vi "Dashboard Main.vi"() -> ()   [LabVIEW 2015]
uses:
  <vilib>/Utility/miscctls.llb/LVRowAndColumnTypeDef.ctl
  <vilib>/event_ctls.llb/eventvkey.ctl
  <vilib>/Rock Robotics/WPI/Dashboard/WPI_DashboardLogging Global.vi
  <vilib>/Rock Robotics/Network Tables/NT Read Numeric Array.vi
  <vilib>/Utility/config.llb/Write Key (String).vi
  <vilib>/Utility/config.llb/Write Key (I32).vi
  <vilib>/Utility/config.llb/NI_LVConfig.lvlib
panel:
  in  "TCP":refnum<k5>
  in  "Rec Mode":enum32{"Stop", "Record", "Playback"}(radio)
  in  "Vision":u16(ring) items=["Camera Off", "USB Camera SW", "USB Camera HW", "IP Camera"]
  out "Camera IP":string
  out "Image Message":string="Timeout in Camera Communications"
  in  "Dashboard Tab":T1(tab)
  out "Speed Control":dbl(slide) scale=0.0..1.0
  out "Right Encoder":dbl format="%#_3g"
  out "Left Encoder":dbl format="%#_3g"
  in  "Autonomous Selection":string(combo)
  out "NT Connection":bool
  in  "Camera Settings":T2={"Frame Rate"=30, "Compression"=30, "Size"=1} {"Frame Rate" scale=1.0..30.0; "Size" items=["640x480", "320x240", "160x120"]}
  out "MotorChart R":cluster{"Numeric":dbl, "Numeric":dbl}(graph)
  out "MotorChart L":T3(graph)
  out "MotorSliders R":cluster{"MotorSlide1":dbl, "MotorSlide2":dbl} {"MotorSlide2" scale=-1.0..1.0 scale format="%#_2e"; "MotorSlide1" scale=-1.0..1.0 scale format="%#_2e"}
  out "MotorSliders L":T4 {"MotorSlide4 2" scale=0.0..14.0 scale format="%#_2e"; "MotorSlide2" scale=-1.0..1.0 scale format="%#_2e"; "MotorSlide1" scale=-1.0..1.0 scale format="%#_2e"}
  out "Gyro":dbl(knob) scale=0.0..360.0
  out "JS1 Z":dbl(slide) scale=-1.0..1.0 scale format="%#_2e"
  out "JS1 Graph":cluster{"X":dbl, "Y":dbl}[](graph)
  out "JS1 Buttons":T5
  out "JS2 Z":dbl(slide) scale=-1.0..1.0 scale format="%#_2e"
  out "JS2 Graph":cluster{"X":dbl, "Y":dbl}[](graph)
  out "JS2 Buttons":T5
  out "Mode":T6(ring)=enum."Auto Disabled"
  in  "DB Camera Config":bool
  out "fps":dbl format="%#.1g"
  out "Mbps":dbl format="%#.1g"
  out "Mbps LED":bool
  out "POV Position":dbl format="%#_3g"
  in  "DB/String 9":string
  in  "DB/String 8":string
  in  "DB/String 7":string
  in  "DB/String 6":string
  in  "DB/String 5":string
  in  "DB/String 4":string
  in  "DB/String 3":string
  in  "DB/String 2":string
  in  "DB/String 1":string
  in  "DB/String 0":string
  in  "DB/Slider 0":dbl(slide) scale=0.0..5.0
  in  "DB/Slider 1":dbl(slide) scale=0.0..5.0
  in  "DB/Slider 2":dbl(slide) scale=0.0..5.0
  in  "DB/Slider 3":dbl(slide) scale=0.0..5.0
  out "DB/LED 3":bool
  out "DB/LED 2":bool
  out "DB/LED 1":bool
  out "DB/LED 0":bool
  in  "DB/Button 3":bool
  in  "DB/Button 2":bool
  in  "DB/Button 1":bool
  in  "DB/Button 0":bool caption="New Name"
  in  "Test Slider":dbl(slide) scale=0.0..100.0 scale format="%#_3g"
  in  "On/Off":bool caption="Solenoid"
  in  "Test Name":u16(ring) items=["Select the test to run..."]
  in  "Test Tree":string(tree)
  in  "Motor":cluster{"Value":dbl, "Enable":bool} {"Value" scale=-1.0..1.0 scale format="%#_3g"}
  out "Progress":T7 {"Test Progress" scale=0.0..100.0}
  in  "Rev/Fwd":cluster{"Forward":bool, "Reverse":bool}
  in  "Test Ring":u16(ring) items=["Monochrome", "Color"]
  out "Cmd Status":string
  in  "Execute Command":bool
  in  "Command Params":string[][](table)
  in  "Command Selection":i32(listbox)
  in  "CheckList":i32(listbox)
  out "Tree":string(tree)
  out "Camera Image":T8(plugin-control)
  out "Background":bool
  # "Left"
  # "Front"
  # "Right"
  # "Battery"
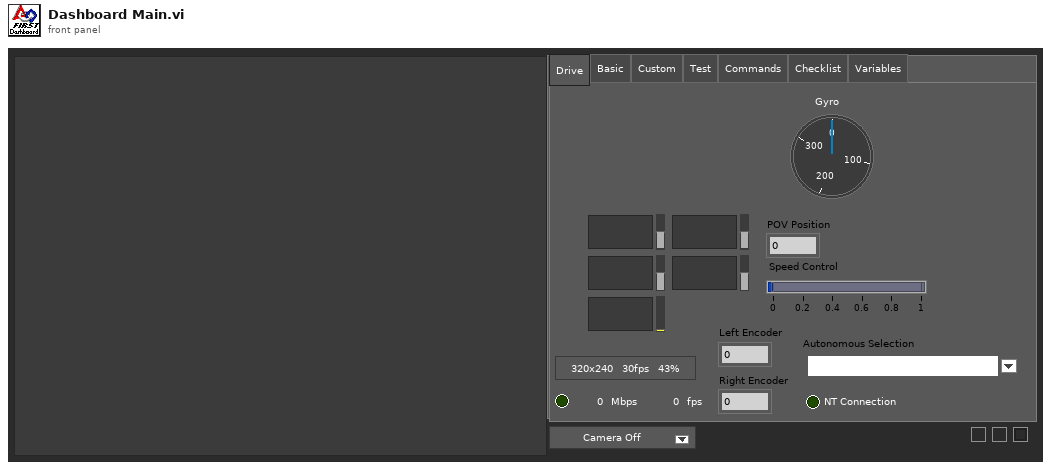
[diagram p1: front panel]
types:
  T1 = enum32{"Drive", "Basic", "Custom", "Test", "Commands", "Checklist", "Variables"}
  T2 = cluster{"Frame Rate":i32, "Compression":i32, "Size":u16}
  T3 = cluster{"Numeric":dbl, "Numeric":dbl, "Battery V":dbl}
  T4 = cluster{"MotorSlide1":dbl, "MotorSlide2":dbl, "MotorSlide4 2":dbl}
  T5 = cluster{bool, bool, bool, bool, bool, bool, bool, bool, bool, bool, bool, bool}
  T6 = enum8{"Tele-Op Disabled", "Tele-Op Enabled", "Auto Disabled", "Auto Enabled", "Test Disabled", "Test Enabled", "Disconnected", "No Code", "E-Stop"}
  T7 = cluster{"Test Progress":u8, "Test Progress Text":string}
  T8 = typedef "IMAQ Image.ctl" = refnum<image>
  T9 = cluster{"IDs":cluster{"RPC field ID":u16, "Unique ID":u16}, "String":string}
  T10 = enum32{"Drive", "Basic", "Custom", "Test", "Checklist", "Variables"}
  T11 = typedef "Image Type" = u32
  T12 = cluster{"Camera Image":refnum<vi>, "Dashboard Tab":refnum<vi>, "Background":refnum<vi>, "Vision":refnum<vi>, "Rec Mode":refnum<vi>, "Test Slider":refnum<vi>, "On/Off ":refnum<vi>, "Test Ring":refnum<vi>, "Rev/Fwd":refnum<vi>, "Test Name":refnum<vi>, "Motor":refnum<vi>, "Progress":refnum<vi>, "CheckList":refnum<vi>, "Tree":refnum<vi>, "Test Tree":refnum<vi>, "Command Params":refnum<vi>, "Command Selection":refnum<vi>, "Execute Command":refnum<vi>, "Cmd Status":refnum<vi>}
  T13 = cluster{"Error Strings":string, "Disable Counts":cluster{u16, u16}, "Rail Faults":cluster{u16, u16, u16}, "Robot IP":string, "DB Mode":u8, "Event Info":cluster{"Name":string, "Type":u8, "Number":u16, "Replay":u8}, "Camera Addr":string}
  T14 = cluster{"Storage":cluster{"Disk Free":u64, "RAM Block":u32, "RAM free":u32}, "CPU Utilization":cluster{"CPU % ISR":sgl, "CPU % Time Crit":sgl, "CPU % Timed Str":sgl, "CPU % High":sgl, "CPU % Above":sgl, "CPU % Normal":sgl, "CPU % Low":sgl}, "CAN":cluster{"% Bus Utilization":sgl, "Bus Off Cnt":u32, "TX_FIFO Full Cnt":u32, "Receive Error Cnt":u8, "Transmit Error Cnt":u8}, "HID":cluster{"HID Outputs":u32, "Rumble Low":u16, "Rumble High":u16}[]}
  T15 = cluster{"Status bits":cluster{"Test Mode":bool, "Autonomous":bool, "Enabled":bool, "Code Start":bool, "Brownout":bool, "Reserved 2":bool, "Reserved 3":bool, "E-Stop":bool}, "Code Trace":cluster{"Disabled":bool, "TeleOp":bool, "Auto":bool, "Test":bool}, "Controller Type":enum16{"unknown", "cRIO", "roboRio"}, "Code?":enum16{"unknown", "noCode", "code"}, "Battery V":dbl}
  T16 = cluster{"Control Bits":cluster{"TestMode":bool, "Autonomous":bool, "Enabled":bool, "FMS Present":bool, bool, bool, bool, "E-Stop":bool}, "Team Station ":u8, "Countdown":sgl, "Joystick Values":cluster{"Axes":dbl[], "Buttons":bool[], "POVs":i16[]}[]}
  T17 = cluster{"Axes":dbl[], "Buttons":bool[], "POVs":i16[]}[]
  T18 = cluster{"Axes":dbl[], "Buttons":bool[], "POVs":i16[]}
  T19 = cluster{"Buttons[0]":bool, "Buttons[1]":bool, "Buttons[2]":bool, "Buttons[3]":bool, "Buttons[4]":bool, "Buttons[5]":bool, "Buttons[6]":bool, "Buttons[7]":bool, "Buttons[8]":bool, "Buttons[9]":bool, "Buttons[10]":bool, "Buttons[11]":bool}
  T20 = typedef "NI_LVConfig.lvlib/Config Data RefNum.ctl" = refnum<k1>
  T21 = cluster{"Operation":enum16{"Update", "Clear"}, "Color Box":u32}[]
  T22 = typedef "eventvkey.ctl" = enum16{"ASCII", "Enter", "Return", "Shift", "Ctrl", "Alt", "Cmd", "Opt", "Caps", "NumLock", "Clear", "Break", "Up", "Down", "Left", "Right", "Insert", "Delete", "Home", "End", "PageUp", "PageDown", "Escape", "Help", "Pause", "ScrollLock", "F1", "F2", "F3", "F4", "F5", "F6", "F7", "F8", "F9", "F10", "F11", "F12", "F13", "F14", "F15", "F16", "F17", "F18", "F19", "F20", "F21", "F22", "F23", "F24", "Play", "VolumeUp", "VolumeDown", "Mute", "Two Byte Char"}
  T23 = cluster{"Image Size":bool, "Image Type":bool, "Pixel Value":bool, "ROI Information":bool, "Zoom Factor":bool}
  T24 = enum8{"Enabled", "Disabled", "Disabled and Grayed Out"}
  T25 = cluster{"Operation":enum16{"Update", "Clear"}, "Color Box":u32}
  T26 = typedef "LVRowAndColumnTypeDef.ctl" = cluster{"Row":i32, "Column":i32}
  T27 = cluster{"Shift":bool, "Ctrl":bool, "Alt":bool, "Cmd":bool, "Opt":bool}
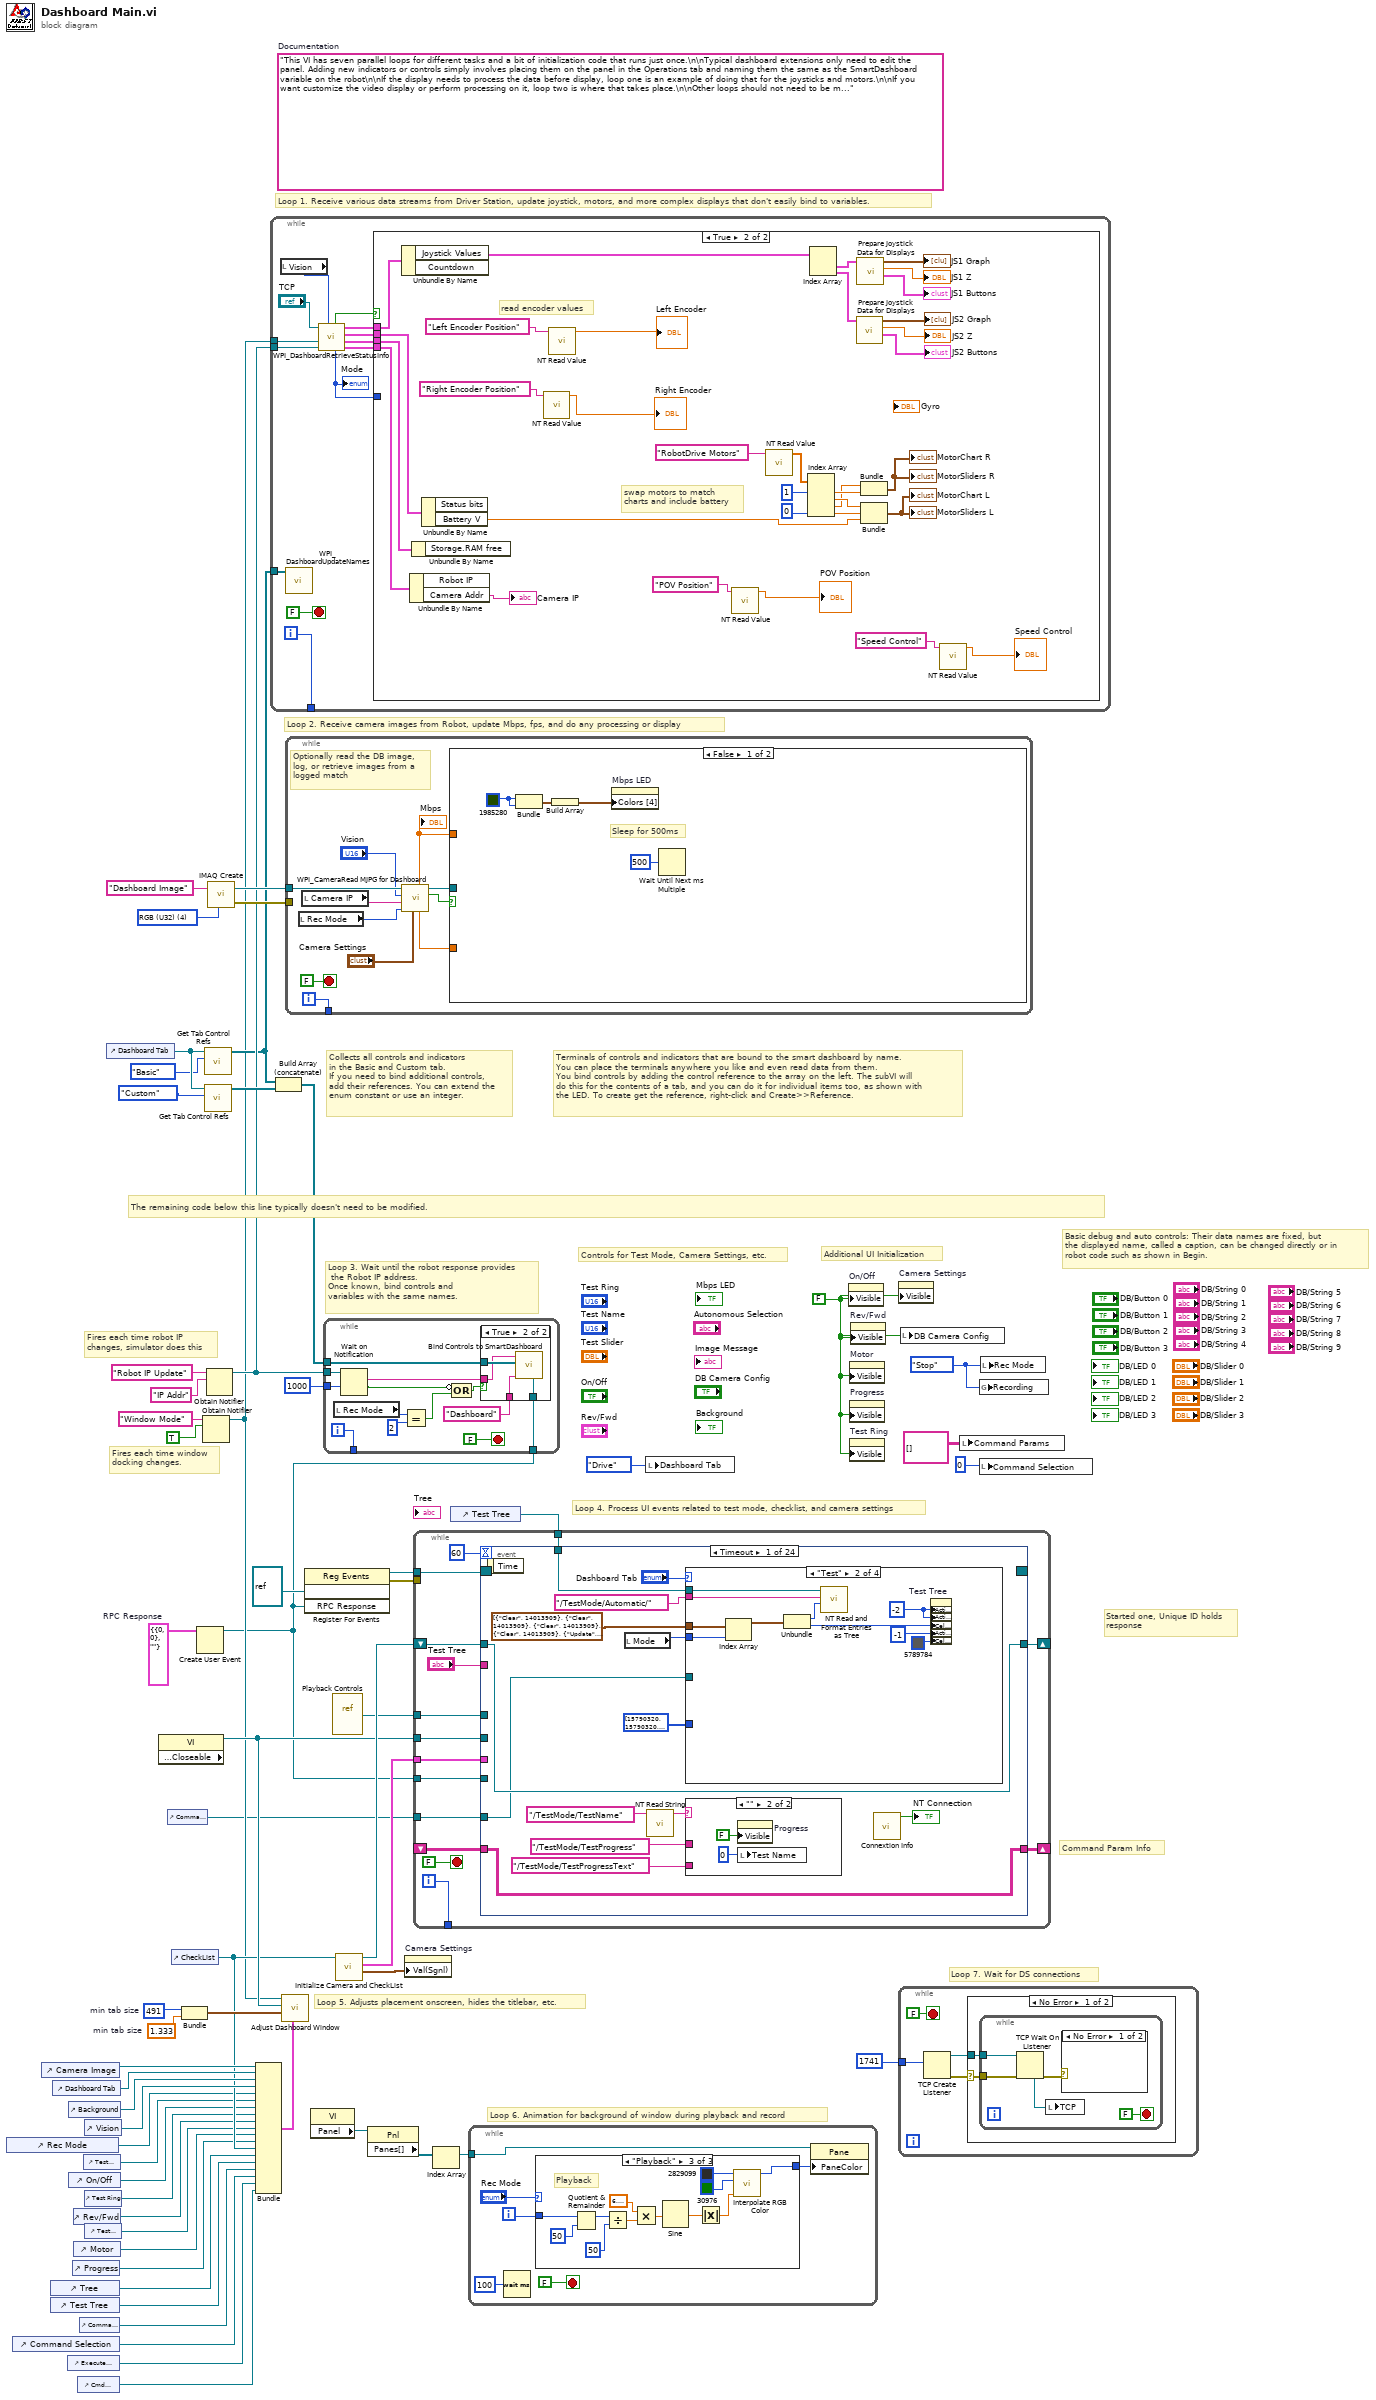
[diagram p0: block diagram]
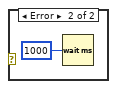
[diagram p2: hidden frame]
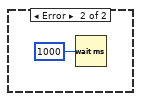
[diagram p3: hidden frame]
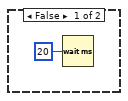
[diagram p4: hidden frame]
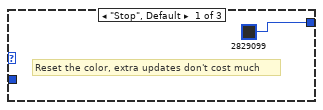
[diagram p5: hidden frame]
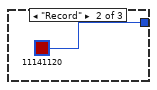
[diagram p6: hidden frame]
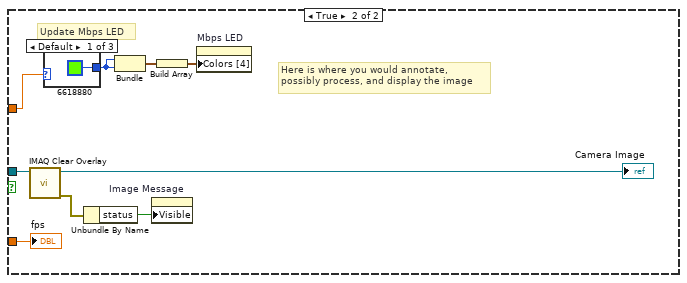
[diagram p8: hidden frame]
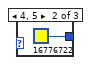
[diagram p9: hidden frame]
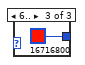
[diagram p10: hidden frame]
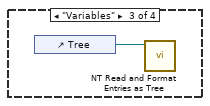
[diagram p12: hidden frame]
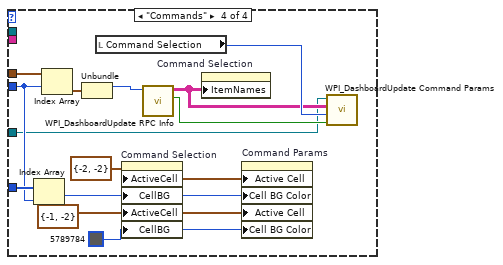
[diagram p13: hidden frame]
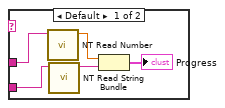
[diagram p14: hidden frame]
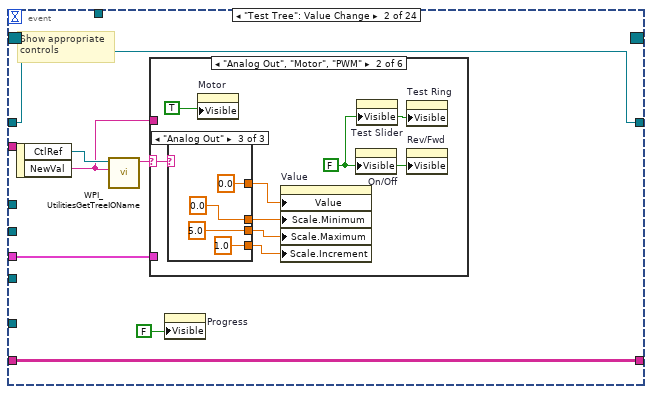
[diagram p15: hidden frame]
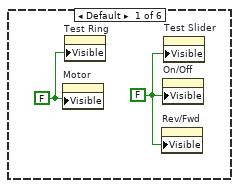
[diagram p16: hidden frame]
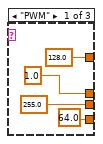
[diagram p17: hidden frame]
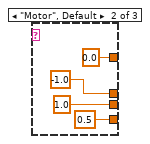
[diagram p18: hidden frame]
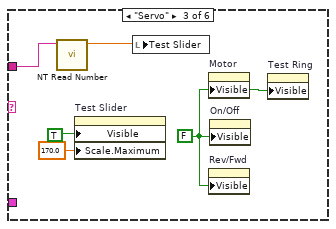
[diagram p19: hidden frame]
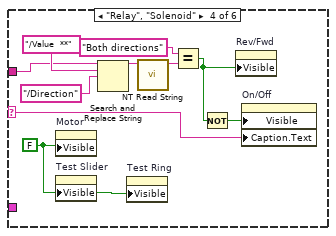
[diagram p20: hidden frame]
diagram:
  w7 = T9 {"IDs"={"RPC field ID"=0, "Unique ID"=0}, "String"=""}  # RPC Response
  w33 = 491  # min tab size
  w32 = 1.333  # min tab size
  w41 = enum32{"Stop", "Record", "Playback"}."Stop" ("Rec Mode")
  w15 = FALSE ("Visible")
  (unwired) "This VI has seven parallel loops for different tasks and a bit of initialization code that runs just once.\n\nTypical dashboard extensions only need to edit the panel. Adding new indicators or controls simply involves placing them on the panel in the Operations tab and naming them the same as the SmartDashboard variable on the robot\n\nIf the display needs to process the data before display, loop one is an example of doing that for the joysticks and motors.\n\nIf you want customize the video display or perform processing on it, loop two is where that takes place.\n\nOther loops should not need to be modified. They are pretty standard, and document the task they perform."  # Documentation
  w61 = T11 4 items=["Grayscale (U8)", "Grayscale (I16)", "Grayscale (SGL)", "Complex (CSG)", "RGB (U32)", "HSL (U32)", "RGB (U64)"] ("Image Type")
  # "Command Param Info"
  # "Started one, Unique ID holds\nresponse"
  # "Loop 7. Wait for DS connections"
  # "Basic debug and auto controls: Their data names are fixed, but\nthe displayed name, called a caption, can be changed directly or in\nrobot code such as shown in Begin."
  # "Controls for Test Mode, Camera Settings, etc."
  # "Additional UI Initialization"
  # "Loop 6. Animation for background of window during playback and record"
  # "Fires each time robot IP\nchanges, simulator does this"
  # "Fires each time window\ndocking changes."
  # "Collects all controls and indicators\nin the Basic and Custom tab.\nIf you need to bind additional controls,\nadd their references. You can extend the\nenum constant or use an integer."
  # "The remaining code below this line typically doesn't need to be modified."
  # "Loop 4. Process UI events related to test mode, checklist, and camera settings"
  # "Terminals of controls and indicators that are bound to the smart dashboard by name.\nYou can place the terminals anywhere you like and even read data from them.\nYou bind controls by adding the control reference to the array on the left. The subVI will\ndo this for the contents of a tab, and you can do it for individual items too, as shown with\nthe LED. To create get the reference, right-click and Create>>Reference."
  # "Loop 3. Wait until the robot response provides\n the Robot IP address.\nOnce known, bind controls and\nvariables with the same names."
  # "Loop 5. Adjusts placement onscreen, hides the titlebar, etc."
  # "Loop 1. Receive various data streams from Driver Station, update joystick, motors, and more complex displays that don't easily bind to variables."
  # "Loop 2. Receive camera images from Robot, update Mbps, fps, and do any processing or display"
  n1 = control-ref of="Rec Mode"() -> (w21:refnum<vi>)
  n2 = control-ref of="Command Selection"() -> (w6:refnum<vi>)
  n3 = control-ref of="Camera Image"() -> (w36:refnum<vi>)
  n4 = control-ref of="Tree"() -> (w25:refnum<vi>)
  n5 = control-ref of="Test Tree"() -> (w24:refnum<vi>)
  n6 = control-ref of="Dashboard Tab"() -> (w35:refnum<vi>)
  n7 = control-ref of="Execute Command"() -> (w8:refnum<vi>)
  n8 = control-ref of="Background"() -> (w30:refnum<vi>)
  n9 = control-ref of="On/Off"() -> (w19:refnum<vi>)
  n10 = control-ref of="Progress"() -> (w16:refnum<vi>)
  n11 = control-ref of="Rev/Fwd"() -> (w17:refnum<vi>)
  n12 = control-ref of="Motor"() -> (w22:refnum<vi>)
  n13 = control-ref of="Cmd Status"() -> (w2:refnum<vi>)
  n14 = control-ref of="Command Params"() -> (w9:refnum<vi>)
  n15 = control-ref of="Test Slider"() -> (w20:refnum<vi>)
  n16 = control-ref of="Vision"() -> (w34:refnum<vi>)
  n17 = control-ref of="Test Ring"() -> (w18:refnum<vi>)
  n18 = control-ref of="Test Name"() -> (w23:refnum<vi>)
  n19 = control-ref of="Dashboard Tab"() -> (w39:refnum<vi>)
  n20 = property class="VI" props=["Front Panel.Closeable"]() -> (reference out=w40:refnum<vi>)  [unwired: 2 in, 2 out]
  n21 = control-ref of="Command Params"() -> (w1:refnum<vi>)
  n22 = control-ref of="CheckList"() -> (w26:refnum<vi>)
  n23 = Bundle("min tab size"=w33, "min tab size"=w32) -> (w31:cluster{"min tab size":i32, "min tab size":dbl})  [unwired: 1 in]
  n24 = Create User Event(user event datatype=w7) -> (user event=w3:refnum<user-event>)  [unwired: 1 in, 1 out]
  n25 = Obtain Notifier(name (unnamed)="Window Mode", notification data type=TRUE) -> (notifier out=w12:refnum<notifier>)  [unwired: 2 in, 2 out]
  n26 = call <vilib>:"Get Tab Control Refs.vi"("Page Index"=T10."Basic" ("Dashboard Tab"), "TabControl in"=w39) -> ("ControlsOnPage"=w13:refnum<vi>[])  [unwired: 9 in]
  n27 = call <vilib>:"Get Tab Control Refs.vi"("Page Index"=T10."Custom" ("Dashboard Tab"), "TabControl in"=w39) -> ("ControlsOnPage"=w38:refnum<vi>[])  [unwired: 9 in]
  n28 = Obtain Notifier(name (unnamed)="Robot IP Update", notification data type="IP Addr" ("name (unnamed)")) -> (notifier out=w14:refnum<notifier>)  [unwired: 2 in, 2 out]
  n29 = call "IMAQ Create"("Image Name"="Dashboard Image", "Image Type"=w61) -> ("New Image"=w59:T8, "error out"=w58:errorcluster)  [unwired: 2 in, 1 out]
  n30 = Bundle("Camera Image"=w36, "Dashboard Tab"=w35, "Background"=w30, "Vision"=w34, "Rec Mode"=w21, "Test Slider"=w20, "On/Off"=w19, "Test Ring"=w18, "Rev/Fwd"=w17, "Test Name"=w23, "Motor"=w22, "Progress"=w16, "CheckList"=w26, "Tree"=w25, "Test Tree"=w24, "Command Params"=w9, "Command Selection"=w6, "Execute Command"=w8, "Cmd Status"=w2) -> (w27:T12)  [unwired: 1 in]
  n31 = while {
    tunnel: [w73] -> _
    tunnel: w14 -> [w67]
    tunnel: w13 -> [w66]
    tunnel: w12 -> [w62]
    i -> [w73]
    stop <- FALSE stop-if-true
    n32 = local read "Vision"() -> (w64:u16)
    n33 = call <vilib>:"WPI_DashboardUpdateNames.vi"("Controls on Tab"=w66) -> ()  [unwired: 11 in]
    n34 = call <vilib>:"WPI_DashboardRetrieveStatusInfo.vi"("Vision"=w64, "Binding Refnum"=w67, "Window Mode Notifier"=w62, "TCP Cnx"="TCP") -> ("Power and Errors"=w68:T13, "Robot Metrics"=w71:T14, "Status Info"=w72:T15, "Control Info"=w69:T16, "Robot Mode"=w65:T6, "Process?"=w70:bool)  [unwired: 2 in]
    "Mode" <- w65
    n35 = case shown="True" w70 {
      tunnel: w72 -> [_ w108]
      tunnel: w71 -> [_ w107]
      tunnel: w69 -> [_ w106]
      tunnel: w68 -> [_ w105]
      tunnel: w65 -> [_ _]
      frame False {
        n36 = Wait (ms)(milliseconds to wait=u32 20) -> ()  [unwired: 1 out]
      }
      frame True {
        # "read encoder values"
        # "swap motors to match\ncharts and include battery"
        n37 = Unbundle By Name(w106) -> ("Joystick Values"=w95:T17)  [unwired: 1 out]
        n38 = Unbundle By Name(w105) -> ("Camera Addr"=→"Camera IP":string)  [unwired: 1 out]
        n39 = Unbundle By Name(w107) -> ()  [unwired: 1 out]
        n40 = Unbundle By Name(w108) -> ("Battery V"=w96:dbl)  [unwired: 1 out]
        n41 = call-poly <vilib>:"NT Read Value.vi"("Name"="Right Encoder Position") -> ("Numeric"=→"Right Encoder":dbl)  [unwired: 9 in, 1 out]
        n42 = call-poly <vilib>:"NT Read Value.vi"("Name"="Left Encoder Position") -> ("Numeric"=→"Left Encoder":dbl)  [unwired: 9 in, 1 out]
        n43 = call-poly <vilib>:"NT Read Value.vi"("Name"="POV Position") -> ("Numeric"=→"POV Position":dbl)  [unwired: 9 in, 1 out]
        n44 = call-poly <vilib>:"NT Read Value.vi"("Name"="RobotDrive Motors") -> ("Numeric Array"=w84:dbl[])  [unwired: 9 in, 1 out]
        n45 = Index Array(array=w84, index #1=1, index #4=0) -> (element #1=w100:dbl, element #2=w101:dbl, element #3=w99:dbl, element #4=w104:dbl)  [unwired: 2 in]
        n46 = Index Array(array=w95) -> (element #1=w94:T18, element #2=w89:T18)  [unwired: 2 in]
        n47 = call "Prepare Joystick Data for Displays.vi"("Joystick Values"=w89) -> ("Buttons"=→"JS2 Buttons":T19, "Z Axis"=→"JS2 Z":dbl, "Cartesian Data"=→"JS2 Graph":cluster{"X axis":dbl, "X axis":dbl}[])  [unwired: 8 in]
        n48 = call "Prepare Joystick Data for Displays.vi"("Joystick Values"=w94) -> ("Buttons"=→"JS1 Buttons":T19, "Z Axis"=→"JS1 Z":dbl, "Cartesian Data"=→"JS1 Graph":cluster{"X axis":dbl, "X axis":dbl}[])  [unwired: 8 in]
        n49 = Bundle("Numeric"=w99, "Numeric"=w100) -> (→"MotorChart R" →"MotorSliders R":cluster{"Numeric":dbl, "Numeric":dbl})  [unwired: 1 in]
        n50 = Bundle("Numeric"=w101, "Numeric"=w104, "Battery V"=w96) -> (→"MotorChart L" →"MotorSliders L":T3)  [unwired: 1 in]
        n51 = call-poly <vilib>:"NT Read Value.vi"("Name"="Speed Control") -> ("Numeric"=→"Speed Control":dbl)  [unwired: 9 in, 1 out]
      }
    }
  }
  n52 = Build Array (concatenate)(w13, w38) -> (w37:refnum<vi>[])
  n53 = call "Adjust Dashboard Window.vi"("Sizing Refnums"=w27, "Size Constraints"=w31, "VI"=w40, "WIn Mode"=w12) -> ()  [unwired: 8 in]
  n54 = while {
    tunnel: w59 -> [w117]
    tunnel: w58 -> [_]
    tunnel: [w118] -> _
    i -> [w118]
    stop <- FALSE stop-if-true
    # "Optionally read the DB image,\nlog, or retrieve images from a\nlogged match"
    n55 = local read "Rec Mode"() -> (w112:enum32{"Stop", "Record", "Playback"})
    n56 = local read "Camera IP"() -> (w110:string)
    n57 = call <vilib>:"WPI_CameraRead MJPG for Dashboard.vi"("Camera Settings"="Camera Settings", "Rec Mode"=w112, "Camera IP"=w110, "Camera Mode"="Vision", "Refnum in"=w117) -> ("Active"=w115:bool, "Refnum out"=w116:T8, "FPS"=w114:dbl, "Bandwidth (Mbps)"=w109:dbl)  [unwired: 3 in]
    "Mbps" <- w109
    n58 = case shown="False" w115 {
      tunnel: w116 -> [_ w127]
      tunnel: w109 -> [_ w126]
      tunnel: w114 -> [_ w124]
      frame False {
        w120 = u32 1985280 ("Color Box")
        # "Sleep for 500ms"
        n59 = Bundle("Color Box"=w120, "Color Box"=w120) -> (w122:cluster{"Color Box":u32, "Color Box":u32})  [unwired: 1 out]
        n60 = Build Array(w122) -> (w121:cluster{"Color Box":u32, "Color Box":u32}[])
        n61 = property on="Mbps LED" class="Bool (strict)"("Colors [4]"=w121) -> ()  [unwired: 2 in, 2 out]
        n62 = Wait Until Next ms Multiple(millisecond multiple=u32 500) -> ()  [unwired: 1 out]
      }
      frame True {
        # "Here is where you would annotate,\npossibly process, and display the image"
        # "Update Mbps LED"
        n63 = call "IMAQ Clear Overlay"("Image"=w127) -> ("error out"=w131:errorcluster, "Image Out"=→"Camera Image":T8)  [unwired: 2 in, 7 out]
        n64 = case shown="Default" w126 {
          tunnel: [u32 6618880 ("Color Box") u32 16776722 ("Color Box") u32 16716800 ("Color Box")] -> w128
          frame Default {
          }
          frame 4, 5 {
          }
          frame 6.. {
          }
        }
        n65 = Unbundle By Name(w131) -> ("status"=w132:bool)
        n66 = Bundle("Color Box"=w128, "Color Box"=w128) -> (w130:cluster{"Color Box":u32, "Color Box":u32})  [unwired: 1 out]
        n67 = property on="Image Message" class="Str"("Visible"=w132) -> ()  [unwired: 2 in, 2 out]
        n68 = Build Array(w130) -> (w129:cluster{"Color Box":u32, "Color Box":u32}[])
        n69 = property on="Mbps LED" class="Bool (strict)"("Colors [4]"=w129) -> ()  [unwired: 2 in, 2 out]
        "fps" <- w124
      }
    }
  }
  n70 = register-events(refnum<vi> refnum, w3) -> (reference out=w45:refnum<event-registration>, error out=w44:errorcluster)  [unwired: 2 in]
  n71 = property class="VI"() -> ("Panel"=w48:refnum<vi>)  [unwired: 2 in, 2 out]
  n72 = while {
    tunnel: w37 -> [w148]
    tunnel: w14 -> [w146]
    tunnel: [w144] -> _
    tunnel: u32 1000 ("milliseconds to wait") -> [w143]
    tunnel: w3 -> [w136]
    i -> [w144]
    stop <- FALSE stop-if-true
    n73 = local read "Rec Mode"() -> (w139:enum32{"Stop", "Record", "Playback"})
    n74 = Wait on Notification(notifier=w146, timeout in ms (-1)=w143) -> (notification=w145:string, timed out?=w141:bool)  [unwired: 2 in, 2 out]
    n75 = Equal?(x=w139, y=u16 2 ("Rec Mode")) -> (x = y?=w140:bool)
    n76 = Compound Arithmetic op=OR(invert w141, w140) -> (w142:bool)
    n77 = case shown="True" w142 {
      tunnel: w148 -> [_ w152]
      tunnel: w145 -> [_ w151]
      tunnel: "Dashboard" -> [_ w150]
      tunnel: w136 -> [_ w149]
      frame False {
      }
      frame True {
        n78 = call <vilib>:"Bind Controls to SmartDashboard.vi"("RPC ref"=w149, "Client Name"=w150, "Bound Control Refs"=w152, "Server IP Address"=w151) -> ()  [unwired: 8 in]
      }
    }
  }
  n79 = vi-ref "Playback Controls.vi"() -> (w46:refnum<vi>)
  n80 = call "Initialize Camera and CheckList.vi"("ListBox in"=w26) -> ("Cluster"=w52:cluster{"value":i32, "value":i32, "index":i32}, "Array"=w53:cluster{string[]}[], "File Refnum"=w51:T20)  [unwired: 8 in]
  n81 = property class="Pnl"(reference=w48) -> ("Panes[]"=w49:refnum<vi>[])  [unwired: 1 in, 2 out]
  n82 = property on="Camera Settings" class="Clust (strict)"("Val(Sgnl)"=w52) -> ()  [unwired: 2 in, 2 out]
  n83 = Index Array(array=w49) -> (element=w47:refnum<vi>)  [unwired: 1 in]
  n84 = control-ref of="Test Tree"() -> (w50:refnum<vi>)
  n85 = while {
    tunnel: w53 -> [w164]
    shift-right: [w163] -> _
    shift-left: w51 -> [w162]
    tunnel: [w161] -> _
    tunnel: w50 -> [w160]
    tunnel: w46 -> [w159]
    tunnel: w45 -> [w158]
    tunnel: w44 -> [_]
    tunnel: w40 -> [w157]
    tunnel: w3 -> [w156]
    tunnel: w1 -> [w155]
    shift-right: [w154] -> _
    shift-left: _ -> [w153]
    i -> [w161]
    stop <- FALSE stop-if-true
    n86 = event shown="[0] Timeout" {
      selector: w158 -> [_ _ _ _ _ _ _ _ _ _ _ _ _ _ _ _ _ _ _ _ _ _ _ _]
      dyn-events: [_ _ _ _ _ _ _ _ _ _ _ _ _ _ _ _ _ _ w473 _ _ _ _ _] -> _
      timeout: u32 60 ("milliseconds to wait") -> [_ _ _ _ _ _ _ _ _ _ _ _ _ _ _ _ _ _ _ _ _ _ _ _]
      tunnel: w160 -> [w177 _ _ _ _ _ _ _ _ _ _ _ _ _ _ _ _ _ _ _ _ _ _ _]
      tunnel: "Test Tree" -> [_ _ _ _ _ _ _ _ _ _ _ _ _ w436 w445 w448 w453 w462 _ _ _ _ _ _]
      tunnel: w164 -> [_ w215 _ _ _ _ _ _ _ _ _ w398 w429 _ _ _ _ _ _ _ _ _ _ _]
      tunnel: [w174 w214 w318 w324 w334 w338 w344 w356 w364 w370 w383 w397 w422 w435 w443 w447 w452 w461 w475 w491 w493 w501 w512 w517] -> w163
      tunnel: w162 -> [w174 w214 w318 w324 w334 w338 w344 w356 w364 w370 w383 w396 w422 w435 w443 w447 w452 w461 w475 w491 w493 w501 w512 w517]
      tunnel: w159 -> [_ _ _ _ _ _ _ _ _ _ _ _ _ _ _ _ _ _ w476 _ w496 _ _ _]
      tunnel: w157 -> [_ _ _ _ _ _ _ _ _ _ _ _ _ _ _ _ _ _ w471 _ _ _ _ _]
      tunnel: w156 -> [_ _ _ _ _ _ _ _ _ _ _ _ _ _ _ _ _ _ w467 _ _ _ _ _]
      tunnel: w155 -> [w169 _ _ _ _ _ w342 _ _ _ _ _ _ _ _ _ _ _ _ _ _ _ _ _]
      tunnel: [w168 w213 w317 w323 w333 w339 w340 w350 w361 w369 w382 w395 w421 w434 w442 w446 w451 w460 w466 w489 w492 w497 w505 w518] -> w154
      tunnel: w153 -> [w168 w213 w317 w323 w333 w339 w340 _ _ w369 w382 w395 w421 w434 w442 w446 w451 w460 w466 w489 w492 w497 w505 w518]
      event Timeout {
        n87 = event-data() -> ()  [unwired: 1 in, 1 out]
        n88 = local read "Mode"() -> (w171:T6)
        n89 = call <vilib>:"NT Read String.vi"("Name"="/TestMode/TestName") -> ("String"=w180:string)  [unwired: 9 in, 1 out]
        n90 = case shown="\"Test\"" "Dashboard Tab" {
          tunnel: w177 -> [_ w191 _ _]
          tunnel: "/TestMode/Automatic/" ("Name Pattern") -> [_ w190 _ _]
          tunnel: T21 [{"Operation"=enum."Clear", "Color Box"=14013909}, {"Operation"=enum."Clear", "Color Box"=14013909}, {"Operation"=enum."Clear", "Color Box"=14013909}, {"Operation"=enum."Clear", "Color Box"=14013909}, {"Operation"=enum."Update", "Color Box"=14013909}, {"Operation"=enum."Update", "Color Box"=16777215}, {"Operation"=enum."Clear", "Color Box"=14013909}, {"Operation"=enum."Clear", "Color Box"=14013909}, {"Operation"=enum."Clear", "Color Box"=14013909}] -> [_ w183 _ w200]
          tunnel: w171 -> [_ w182 _ w199]
          tunnel: u32[] [15790320, 15790320, 15790320, 15790320, 16777215, 16777215, 15790320, 15790320, 15790320] -> [_ _ _ w205]
          tunnel: w169 -> [_ _ _ w193]
          frame "Custom", Default {
          }
          frame "Test" {
            w189 = -2 ("Active Item:Row Number")
            n91 = Index Array(array=w183, index=w182) -> (element=w184:T25)
            n92 = Unbundle(w184) -> ("Operation"=w185:enum16{"Update", "Clear"}, "Color Box"=w186:u32)
            n93 = call <vilib>:"NT Read and Format Entries as Tree.vi"("Operation"=w185, "Name Pattern"=w190, "Tree Refnum"=w191) -> ()  [unwired: 7 in, 2 out]
            n94 = property on="Test Tree" class="Tree (strict)"("Active Item Row Number"=w189, "ActiveColNum"=w189, "CellBG"=w186, "Active Item Row Number"=-1 ("Active Item:Row Number"), "CellBG"=u32 5789784 ("Color Box")) -> ()  [unwired: 2 in, 2 out]
          }
          frame "Variables" {
            n95 = control-ref of="Tree"() -> (w192:refnum<vi>)
            n96 = call <vilib>:"NT Read and Format Entries as Tree.vi"("Tree Refnum"=w192) -> ()  [unwired: 9 in, 2 out]
          }
          frame "Commands" {
            w201 = u32 5789784 ("Color Box")
            w202 = T26 {"Row"=-1, "Column"=-2} ("Active Cell:Active Cell")
            w204 = T26 {"Row"=-2, "Column"=-2} ("Active Cell:Active Cell")
            n97 = Index Array(array=w205, index=w199) -> (element=w203:u32)
            n98 = Index Array(array=w200, index=w199) -> (element=w198:T25)
            n99 = Unbundle(w198) -> ("Operation"=w197:enum16{"Update", "Clear"})  [unwired: 1 out]
            n100 = local read "Command Selection"() -> (w196:i32)
            n101 = property on="Command Selection" class="MCListbox (strict)"("ActiveCell"=w204, "CellBG"=w203, "ActiveCell"=w202, "CellBG"=w201) -> ()  [unwired: 2 in, 2 out]
            n102 = call <vilib>:"WPI_DashboardUpdate RPC Info.vi"("Operation"=w197) -> ("update"=w195:bool, "commands"=w194:string[][])  [unwired: 9 in]
            n103 = property on="Command Selection" class="MCListbox (strict)"("ItemNames"=w194) -> ()  [unwired: 2 in, 2 out]
            n104 = property on="Command Params" class="Tbl (strict)"("Active Cell"=w204, "Cell BG Color"=w203, "Active Cell"=w202, "Cell BG Color"=w201) -> ()  [unwired: 2 in, 2 out]
            n105 = call <vilib>:"WPI_DashboardUpdate Command Params.vi"("Update"=w195, "NewVal"=w196, "Commands"=w194, "Param Tbl"=w193) -> ()  [unwired: 7 in, 1 out]
          }
        }
        n106 = case shown="\"\"" w180 {
          tunnel: "/TestMode/TestProgress" ("Name") -> [w207 _]
          tunnel: "/TestMode/TestProgressText" ("Name") -> [w206 _]
          frame Default {
            n107 = call <vilib>:"NT Read Number.vi"("Name"=w207) -> ("Numeric"=w208:dbl)  [unwired: 9 in, 1 out]
            n108 = call <vilib>:"NT Read String.vi"("Name"=w206) -> ("String"=w209:string)  [unwired: 9 in, 1 out]
            n109 = Bundle("Numeric"=w208, "String"=w209) -> (→"Progress":cluster{"Numeric":dbl, "String":string})  [unwired: 1 in]
          }
          frame "" {
            n110 = property on="Progress" class="Clust (strict)"("Visible"=FALSE) -> ()  [unwired: 2 in, 2 out]
            n111 = local write "Test Name"(u16 0) -> ()
          }
        }
        n112 = call <vilib>:"Connextion Info.vi"() -> ("Connected"=→"NT Connection":bool)  [unwired: 10 in, 1 out]
      }
      event "Test Tree": Value Change {
        # "Show appropriate\ncontrols"
        n113 = event-data() -> ("CtlRef"=w218:refnum<vi>, "NewVal"=w216:string)  [unwired: 1 in]
        n114 = call <vilib>:"WPI_UtilitiesGetTreeIOName.vi"("NewVal"=w216, "TreeControl in"=w218) -> ("I/O Name"=w219:string)  [unwired: 9 in]
        n115 = case shown="\"Analog Out\", \"Motor\", \"PWM\"" w219 {
          selector: w219 -> [_ w226 _ w248 w257 _]
          tunnel: w216 -> [_ _ w245 w247 _ w264]
          tunnel: w215 -> [_ _ _ _ _ w263]
          frame Default {
            w221 = FALSE ("Visible")
            w220 = FALSE ("Visible")
            n116 = property on="Motor" class="Clust (strict)"("Visible"=w220) -> ()  [unwired: 2 in, 2 out]
            n117 = property on="Test Ring" class="Ring (strict)"("Visible"=w220) -> ()  [unwired: 2 in, 2 out]
            n118 = property on="Rev/Fwd" class="Clust (strict)"("Visible"=w221) -> ()  [unwired: 2 in, 2 out]
            n119 = property on="On/Off" class="Bool (strict)"("Visible"=w221) -> ()  [unwired: 2 in, 2 out]
            n120 = property on="Test Slider" class="Slide (strict)"("Visible"=w221) -> ()  [unwired: 2 in, 2 out]
          }
          frame "Analog Out", "Motor", "PWM" {
            w227 = FALSE ("Visible")
            n121 = case shown="\"Analog Out\"" w226 {
              tunnel: [1.0 ("Value") -1.0 ("Value") 0.0 ("Value")] -> w225
              tunnel: [255.0 ("Value") 1.0 ("Value") 5.0 ("Value")] -> w224
              tunnel: [128.0 ("Value") 0.0 ("Value") 0.0 ("Value")] -> w223
              tunnel: [64.0 ("Value") 0.5 ("Value") 1.0 ("Value")] -> w222
              frame "PWM" {
              }
              frame "Motor", Default {
              }
              frame "Analog Out" {
              }
            }
            n122 = property on="Motor" class="Clust (strict)"("Visible"=TRUE) -> ()  [unwired: 2 in, 2 out]
            n123 = property on="Value" class="Slide (strict)"("Value"=w223, "Scale.Minimum"=w225, "Scale.Maximum"=w224, "Scale.Increment"=w222) -> ()  [unwired: 2 in, 2 out]
            n124 = property on="On/Off" class="Bool (strict)"("Visible"=w227) -> ()  [unwired: 2 in, 2 out]
            n125 = property on="Test Slider" class="Slide (strict)"("Visible"=w227) -> ()  [unwired: 2 in, 2 out]
            n126 = property on="Test Ring" class="Ring (strict)"("Visible"=w227) -> ()  [unwired: 2 in, 2 out]
            n127 = property on="Rev/Fwd" class="Clust (strict)"("Visible"=w227) -> ()  [unwired: 2 in, 2 out]
          }
          frame "Servo" {
            w243 = FALSE ("Visible")
            n128 = call <vilib>:"NT Read Number.vi"("Name"=w245) -> ("Numeric"=w244:dbl)  [unwired: 9 in, 1 out]
            n129 = property on="Test Slider" class="Slide (strict)"("Visible"=TRUE, "Scale.Maximum"=170.0 ("Scale.Range:Maximum")) -> ()  [unwired: 2 in, 2 out]
            n130 = local write "Test Slider"(w244) -> ()
            n131 = property on="Motor" class="Clust (strict)"("Visible"=w243) -> ()  [unwired: 2 in, 2 out]
            n132 = property on="Rev/Fwd" class="Clust (strict)"("Visible"=w243) -> ()  [unwired: 2 in, 2 out]
            n133 = property on="On/Off" class="Bool (strict)"("Visible"=w243) -> ()  [unwired: 2 in, 2 out]
            n134 = property on="Test Ring" class="Ring (strict)"("Visible"=w243) -> ()  [unwired: 2 in, 2 out]
          }
          frame "Relay", "Solenoid" {
            w246 = FALSE ("Visible")
            n135 = property on="Motor" class="Clust (strict)"("Visible"=w246) -> ()  [unwired: 2 in, 2 out]
            n136 = property on="Test Slider" class="Slide (strict)"("Visible"=w246) -> ()  [unwired: 2 in, 2 out]
            n137 = Search and Replace String(input string=w247, search string="/Value  **", replace string="/Direction") -> (result string=w253:string)  [unwired: 5 in, 3 out]
            n138 = property on="Test Ring" class="Ring (strict)"("Visible"=w246) -> ()  [unwired: 2 in, 2 out]
            n139 = call <vilib>:"NT Read String.vi"("Name"=w253) -> ("String"=w251:string)  [unwired: 9 in, 1 out]
            n140 = Equal?(x="Both directions", y=w251) -> (x = y?=w249:bool)
            n141 = Not(x=w249) -> (.not. x?=w250:bool)
            n142 = property on="Rev/Fwd" class="Clust (strict)"("Visible"=w249) -> ()  [unwired: 2 in, 2 out]
            n143 = property on="On/Off" class="Bool (strict)"("Visible"=w250, "Caption.Text"=w248) -> ()  [unwired: 2 in, 2 out]
          }
          frame "Compressor", "Digital Out" {
            w256 = FALSE ("Visible")
            # "Get direction and finish"
            n144 = property on="Motor" class="Clust (strict)"("Visible"=w256) -> ()  [unwired: 2 in, 2 out]
            n145 = property on="Test Slider" class="Slide (strict)"("Visible"=w256) -> ()  [unwired: 2 in, 2 out]
            n146 = property on="Test Ring" class="Ring (strict)"("Visible"=w256) -> ()  [unwired: 2 in, 2 out]
            n147 = property on="On/Off" class="Bool (strict)"("Visible"=TRUE, "Caption.Text"=w257) -> ()  [unwired: 2 in, 2 out]
            n148 = property on="Rev/Fwd" class="Clust (strict)"("Visible"=FALSE) -> ()  [unwired: 2 in, 2 out]
          }
          frame "Camera" {
            n149 = call <vilib>:"Get Last Path Segment.vi"("String in"=w264) -> ("String out"=w265:string)  [unwired: 10 in]
            n150 = property on="On/Off" class="Bool (strict)"("Visible"=FALSE) -> ()  [unwired: 2 in, 2 out]
            n151 = property on="Motor" class="Clust (strict)"("Visible"=FALSE) -> ()  [unwired: 2 in, 2 out]
            n152 = property on="Rev/Fwd" class="Clust (strict)"("Visible"=FALSE) -> ()  [unwired: 2 in, 2 out]
            n153 = case shown="\"White Balance  **\"" w265 {
              tunnel: w264 -> [w271 w280 w289 w298 w307 _ w313]
              tunnel: w263 -> [w269 w277 w286 w295 w304 _ _]
              frame "Size  **" {
                n154 = Index Array(array=w269) -> (element=w268:cluster{string[]})  [unwired: 1 in]
                n155 = call <vilib>:"NT Read String.vi"("Name"=w271) -> ("String"=w270:string)  [unwired: 9 in, 1 out]
                n156 = Unbundle(w268) -> (w266:string[])
                n157 = Match First String(2:w266, 3:w270) -> (0:w267:i32)  [unwired: 1 out]
                n158 = property on="Test Ring" class="Ring (strict)"("Value"=w267, "Strings []"=w266) -> ()  [unwired: 2 in, 2 out]
                n159 = property on="Test Ring" class="Ring (strict)"("Visible"=TRUE) -> ()  [unwired: 2 in, 2 out]
                n160 = property on="Test Slider" class="Slide (strict)"("Visible"=FALSE) -> ()  [unwired: 2 in, 2 out]
              }
              frame "White Balance  **" {
                n161 = Index Array(array=w277, index=1) -> (element=w278:cluster{string[]})
                n162 = call <vilib>:"NT Read String.vi"("Name"=w280) -> ("String"=w279:string)  [unwired: 9 in, 1 out]
                n163 = Unbundle(w278) -> (w275:string[])
                n164 = Match First String(2:w275, 3:w279) -> (0:w274:i32)  [unwired: 1 out]
                n165 = property on="Test Ring" class="Ring (strict)"("Value"=w274, "Strings []"=w275) -> ()  [unwired: 2 in, 2 out]
                n166 = property on="Test Ring" class="Ring (strict)"("Visible"=TRUE) -> ()  [unwired: 2 in, 2 out]
                n167 = property on="Test Slider" class="Slide (strict)"("Visible"=FALSE) -> ()  [unwired: 2 in, 2 out]
              }
              frame "Exposure  **" {
                n168 = Index Array(array=w286, index=2) -> (element=w287:cluster{string[]})
                n169 = call <vilib>:"NT Read String.vi"("Name"=w289) -> ("String"=w288:string)  [unwired: 9 in, 1 out]
                n170 = Unbundle(w287) -> (w283:string[])
                n171 = Match First String(2:w283, 3:w288) -> (0:w284:i32)  [unwired: 1 out]
                n172 = property on="Test Ring" class="Ring (strict)"("Value"=w284, "Strings []"=w283) -> ()  [unwired: 2 in, 2 out]
                n173 = property on="Test Ring" class="Ring (strict)"("Visible"=TRUE) -> ()  [unwired: 2 in, 2 out]
                n174 = property on="Test Slider" class="Slide (strict)"("Visible"=FALSE) -> ()  [unwired: 2 in, 2 out]
              }
              frame "Exposure Priority  **" {
                n175 = Index Array(array=w295, index=3) -> (element=w296:cluster{string[]})
                n176 = call <vilib>:"NT Read String.vi"("Name"=w298) -> ("String"=w297:string)  [unwired: 9 in, 1 out]
                n177 = Unbundle(w296) -> (w292:string[])
                n178 = Match First String(2:w292, 3:w297) -> (0:w293:i32)  [unwired: 1 out]
                n179 = property on="Test Ring" class="Ring (strict)"("Value"=w293, "Strings []"=w292) -> ()  [unwired: 2 in, 2 out]
                n180 = property on="Test Ring" class="Ring (strict)"("Visible"=TRUE) -> ()  [unwired: 2 in, 2 out]
                n181 = property on="Test Slider" class="Slide (strict)"("Visible"=FALSE) -> ()  [unwired: 2 in, 2 out]
              }
              frame "Color Enable  **" {
                n182 = Index Array(array=w304, index=4) -> (element=w305:cluster{string[]})
                n183 = call <vilib>:"NT Read String.vi"("Name"=w307) -> ("String"=w306:string)  [unwired: 9 in, 1 out]
                n184 = Unbundle(w305) -> (w301:string[])
                n185 = Match First String(2:w301, 3:w306) -> (0:w302:i32)  [unwired: 1 out]
                n186 = property on="Test Ring" class="Ring (strict)"("Value"=w302, "Strings []"=w301) -> ()  [unwired: 2 in, 2 out]
                n187 = property on="Test Ring" class="Ring (strict)"("Visible"=TRUE) -> ()  [unwired: 2 in, 2 out]
                n188 = property on="Test Slider" class="Slide (strict)"("Visible"=FALSE) -> ()  [unwired: 2 in, 2 out]
              }
              frame Default {
                n189 = property on="Test Ring" class="Ring (strict)"("Visible"=FALSE) -> ()  [unwired: 2 in, 2 out]
                n190 = property on="Test Slider" class="Slide (strict)"("Visible"=FALSE) -> ()  [unwired: 2 in, 2 out]
              }
              frame "Brightness  **", "Color Level  **", "Compression  **", "FPS  **", "Sharpness  **" {
                n191 = call <vilib>:"NT Read Number.vi"("Name"=w313) -> ("Numeric"=w312:dbl)  [unwired: 9 in, 1 out]
                n192 = local write "Test Slider"(w312) -> ()
                n193 = property on="Test Slider" class="Slide (strict)"("Visible"=TRUE, "Scale.Maximum"=100.0 ("Scale.Range:Maximum")) -> ()  [unwired: 2 in, 2 out]
                n194 = property on="Test Ring" class="Ring (strict)"("Visible"=FALSE) -> ()  [unwired: 2 in, 2 out]
              }
            }
          }
        }
        n195 = property on="Progress" class="Clust (strict)"("Visible"=FALSE) -> ()  [unwired: 2 in, 2 out]
      }
      event "Test Name": Mouse Enter {
        # "Populate the ring with the list of tests"
        n196 = event-data() -> ()  [unwired: 1 in, 1 out]
        n197 = call <vilib>:"NT Read String Array.vi"("Name"="/TestMode/TestList") -> ("String Array"=w322:string[])  [unwired: 9 in, 1 out]
        n198 = Build Array (concatenate)("Select the test to run...", w322) -> (w321:string[])
        n199 = property on="Test Name" class="Ring (strict)"("Strings []"=w321) -> ()  [unwired: 2 in, 2 out]
      }
      event "Test Name": Value Change {
        w325 = FALSE ("Visible")
        # "Tell the robot the test name to run"
        n200 = event-data() -> ("NewVal"=w329:u16)  [unwired: 1 in]
        n201 = property on="Test Name" class="Ring (strict)"() -> ("Strings []"=w330:string[])  [unwired: 2 in, 2 out]
        n202 = local write "Progress"(T7 {"Test Progress"=0, "Test Progress Text"=""} ("Progress")) -> ()
        n203 = Index Array(array=w330, index=w329) -> (element=w328:string)
        n204 = call <vilib>:"NT Write String.vi"("String"=w328, "Name"="/TestMode/TestName") -> ()  [unwired: 9 in, 1 out]
        n205 = property on="Progress" class="Clust (strict)"("Visible"=TRUE) -> ()  [unwired: 2 in, 2 out]
        n206 = property on="Motor" class="Clust (strict)"("Visible"=w325) -> ()  [unwired: 2 in, 2 out]
        n207 = property on="Test Slider" class="Slide (strict)"("Visible"=w325) -> ()  [unwired: 2 in, 2 out]
        n208 = property on="On/Off" class="Bool (strict)"("Visible"=w325) -> ()  [unwired: 2 in, 2 out]
        n209 = property on="Rev/Fwd" class="Clust (strict)"("Visible"=w325) -> ()  [unwired: 2 in, 2 out]
        n210 = property on="Test Ring" class="Ring (strict)"("Visible"=w325) -> ()  [unwired: 2 in, 2 out]
      }
      event "Autonomous Selection": Mouse Enter {
        # "Populate the combo box with the list of autonomous options"
        n211 = event-data() -> ()  [unwired: 1 in, 1 out]
        n212 = call <vilib>:"NT Read String Array.vi"("Name"="Auto List") -> ("String Array"=w332:string[])  [unwired: 9 in, 1 out]
        n213 = property on="Autonomous Selection" class="CmbBox"("Strings[]"=w332) -> ()  [unwired: 2 in, 2 out]
      }
      event "Autonomous Selection": Value Change {
        # "User modified the Auto Selection. Write to NT variable so robot knows."
        n214 = event-data() -> ("NewVal"=w336:string)  [unwired: 1 in]
        n215 = call <vilib>:"NT Write String.vi"("String"=w336, "Name"="Auto Selector") -> ()  [unwired: 9 in, 1 out]
      }
      event "Command Selection": Value Change {
        # "Get the params and show in table"
        n216 = event-data() -> ("NewVal"=w343:i32)  [unwired: 1 in]
        n217 = property on="Command Selection" class="MCListbox (strict)"() -> ("ItemNames"=w341:string[][])  [unwired: 2 in, 2 out]
        n218 = call <vilib>:"WPI_DashboardUpdate Command Params.vi"("NewVal"=w343, "Commands"=w341, "Param Tbl"=w342) -> ()  [unwired: 8 in, 1 out]
      }
      event "Execute Command": Value Change {
        # "Started one, Unique ID holds\nresponse"
        n219 = event-data() -> ()  [unwired: 1 in, 1 out]
        n220 = property on="Command Selection" class="MCListbox (strict)"() -> ("ItemNames"=w355:string[][])  [unwired: 2 in, 2 out]
        n221 = Index Array(array=w355, index (row)="Command Selection", index (col)=0) -> (element=w353:string)
        n222 = call <vilib>:"Invoke Commands.vi"("Command Params"="Command Params", "Function Name"=w353) -> ("Params"=w349:u8, "Started"=w348:bool)  [unwired: 7 in, 1 out]
        n223 = Array Subset(array="Command Params", length (row)=w349) -> (w350:string[][])  [unwired: 3 in]
        n224 = Select(t="Executing" ("Cmd Status"), s=w348, f="" ("Cmd Status")) -> (s? t:f=→"Cmd Status":string)
      }
      event "Command Selection": Double Click {
        n225 = event-data() -> ("Row"=w365:i32)  [unwired: 1 in]
        n226 = property on="Command Selection" class="MCListbox (strict)"() -> ("ItemNames"=w368:string[][])  [unwired: 2 in, 2 out]
        n227 = local read "Command Params"() -> (w363:string[][])
        n228 = Index Array(array=w368, index (row)=w365, index (col)=0) -> (element=w366:string)
        n229 = call <vilib>:"Invoke Commands.vi"("Command Params"=w363, "Function Name"=w366) -> ("Params"=w362:u8, "Started"=w357:bool)  [unwired: 7 in, 1 out]
        n230 = Array Subset(array=w363, length (row)=w362) -> (w361:string[][])  [unwired: 3 in]
        n231 = Select(t="Executing" ("Cmd Status"), s=w357, f="" ("Cmd Status")) -> (s? t:f=w358:string)
        n232 = local write "Cmd Status"(w358) -> ()
      }
      event "CheckList": Double Click {
        # "Shift clears all"
        # "Update symbols on the listbox"
        n233 = event-data() -> ("PlatMods.Shift"=w371:bool, "Row"=w373:i32)  [unwired: 1 in]
        n234 = case shown="True" w371 {
          tunnel: w373 -> [w377 _]
          tunnel: 1 -> [w376 _]
          frame False {
            n235 = property on="CheckList" class="LstBox (strict)"() -> ("Item Symbols"=w375:i32[])  [unwired: 2 in, 2 out]
            n236 = Replace Array Subset(array=w375, new element=w376, index=w377) -> (w374:i32[])
            n237 = property on="CheckList" class="LstBox (strict)"("Item Symbols"=w374) -> ()  [unwired: 2 in, 2 out]
          }
          frame True {
            w378 = 0 ("Top Row")
            n238 = property on="CheckList" class="LstBox (strict)"() -> ("Number of Rows"=w380:u32)  [unwired: 2 in, 2 out]
            n239 = Initialize Array(0, w380) -> (w379:i32[])
            n240 = property on="CheckList" class="LstBox (strict)"("Top Row"=w378, "Value"=w378, "Item Symbols"=w379) -> ()  [unwired: 2 in, 2 out]
          }
        }
      }
      event "CheckList": Key Down {
        # "Update symbols on the listbox\nLeft and right keys check and uncheck"
        n241 = event-data() -> ("VKey"=w385:T22)  [unwired: 1 in]
        n242 = case shown="\"Left\", \"Right\"" w385 {
          selector: w385 -> [w390 _]
          tunnel: eventvkey."Left" ("VKey") -> [w388 _]
          frame "Left", "Right" {
            n243 = Equal?(x=w388, y=w390) -> (x = y?=w389:bool)
            n244 = Select(t=0, s=w389, f=1) -> (s? t:f=w391:i32)
            n245 = property on="CheckList" class="LstBox (strict)"() -> ("Item Symbols"=w394:i32[])  [unwired: 2 in, 2 out]
            n246 = Replace Array Subset(array=w394, new element=w391, index="CheckList") -> (w393:i32[])
            n247 = property on="CheckList" class="LstBox (strict)"("Item Symbols"=w393) -> ()  [unwired: 2 in, 2 out]
          }
          frame Default {
          }
        }
      }
      event "DB Camera Config": Value Change {
        # "Show or hide the cluster of controls, store in ini file"
        n248 = event-data() -> ("NewVal"=w399:bool)  [unwired: 1 in]
        n249 = case shown="False" w399 {
          tunnel: w398 -> [w408 _]
          tunnel: [w401 w419] -> w397
          tunnel: w396 -> [w400 w419]
          frame False {
            w415 = "Camera"
            w418 = FALSE ("Visible")
            n250 = local read "Camera Settings"() -> (w407:T2)
            n251 = Index Array(array=w408) -> (element=w411:cluster{string[]})  [unwired: 1 in]
            n252 = Unbundle(w407) -> ("Frame Rate"=w406:i32, "Compression"=w405:i32, "Size"=w409:u16)
            n253 = Unbundle(w411) -> (w410:string[])
            n254 = Index Array(array=w410, index=w409) -> (element=w404:string)
            n255 = call-poly <vilib>:"Write Key.vi"("section"=w415, "value"=w404, "key"="Size", "refnum"=w400) -> ("refnum out"=w417:T20)  [unwired: 2 in, 5 out]
            n256 = call-poly <vilib>:"Write Key.vi"("section"=w415, "value"=w406, "key"="FrameRate", "refnum"=w417) -> ("refnum out"=w416:T20)  [unwired: 1 in, 6 out]
            n257 = property on="Camera Settings" class="Clust (strict)"("Visible"=w418) -> ()  [unwired: 2 in, 2 out]
            n258 = local write "DB Camera Config"(w418) -> ()
            n259 = call-poly <vilib>:"Write Key.vi"("section"=w415, "value"=w405, "key"="Compression", "refnum"=w416) -> ("refnum out"=w402:T20)  [unwired: 1 in, 6 out]
            n260 = call <vilib>:"Close Config Data.vi"("refnum"=w402) -> ("file path"=w403:path)  [unwired: 2 in, 8 out]
            n261 = call <vilib>:"Open Config Data.vi"("configuration file path"=w403) -> ("refnum"=w401:T20)  [unwired: 8 in, 2 out]
          }
          frame True {
            n262 = property on="Camera Settings" class="Clust (strict)"("Visible"=TRUE) -> ()  [unwired: 2 in, 2 out]
          }
        }
      }
      event "Camera Settings": Value Change {
        # "Update summary string when any elements of DB camera change"
        n263 = event-data() -> ("NewVal"=w433:T2)  [unwired: 1 in]
        n264 = Index Array(array=w429) -> (element=w428:cluster{string[]})  [unwired: 1 in]
        n265 = Unbundle(w433) -> ("Frame Rate"=w424:i32, "Compression"=w423:i32, "Size"=w426:u16)
        n266 = Unbundle(w428) -> (w427:string[])
        n267 = Index Array(array=w427, index=w426) -> (element=w425:string)
        n268 = Format Into String(format string="%s   %dfps   %d%%", w425, w424, w423) -> (resulting string=w430:string)  [unwired: 2 in, 1 out]
        n269 = Build Array(w430) -> (w431:string[])
        n270 = property on="DB Camera Config" class="Bool (strict)"("Strings [4]"=w431) -> ()  [unwired: 2 in, 2 out]
      }
      event "Motor.Enable": Value Change {
        # "When the test mode otor enable helper is set, update that\ntree row item's value"
        n271 = event-data() -> ("NewVal"=w440:bool)  [unwired: 1 in]
        n272 = Unbundle("Motor") -> ("Value"=w439:dbl)  [unwired: 1 out]
        n273 = Select(t=w439, s=w440, f=0.0) -> (s? t:f=w437:dbl)
        n274 = call <vilib>:"NT Write Number.vi"("Numeric"=w437, "Name"=w436) -> ()  [unwired: 9 in, 1 out]
      }
      event "Test Slider": Value Change {
        # "When the test mode slider helper is set, update that\ntree row item's value"
        n275 = event-data() -> ("NewVal"=w444:dbl)  [unwired: 1 in]
        n276 = call <vilib>:"NT Write Number.vi"("Numeric"=w444, "Name"=w445) -> ()  [unwired: 9 in, 1 out]
      }
      event "On/Off": Value Change {
        # "When the test mode on/off helper value is set, update that\ntree row item's value"
        n277 = event-data() -> ("NewVal"=w450:bool)  [unwired: 1 in]
        n278 = Boolean To (0,1)(Boolean=w450) -> (0, 1=w449:i16)
        n279 = call <vilib>:"NT Write Number.vi"("Numeric"=w449, "Name"=w448) -> ()  [unwired: 9 in, 1 out]
      }
      event "Rev/Fwd": Value Change {
        # "When the test mode helper value for relays is set, update that\ntree row item's value"
        n280 = event-data() -> ("NewVal.Forward"=w459:bool, "NewVal.Reverse"=w458:bool)  [unwired: 1 in]
        n281 = Boolean To (0,1)(Boolean=w459) -> (0, 1=w455:i16)
        n282 = Boolean To (0,1)(Boolean=w458) -> (0, 1=w457:i16)
        n283 = Negate(x=w457) -> (-x=w456:i16)
        n284 = Add(x=w455, y=w456) -> (x+y=w454:i16)
        n285 = call <vilib>:"NT Write Number.vi"("Numeric"=w454, "Name"=w453) -> ()  [unwired: 9 in, 1 out]
      }
      event "Test Ring": Value Change {
        # "When a test mode helper value is selected from the ring,\nset the tree item's variable to the string value"
        n286 = event-data() -> ("NewVal"=w464:u16)  [unwired: 1 in]
        n287 = property on="Test Ring" class="Ring (strict)"() -> ("Strings []"=w465:string[])  [unwired: 2 in, 2 out]
        n288 = Index Array(array=w465, index=w464) -> (element=w463:string)
        n289 = call <vilib>:"NT Write String.vi"("String"=w463, "Name"=w462) -> ()  [unwired: 9 in, 1 out]
      }
      event "Rec Mode": Value Change {
        # "Update globals for recording mode and path to read log from.\nClear when logging and let NetworkTables set path for vision to\nuse."
        n290 = event-data() -> ("NewVal"=w477:enum32{"Stop", "Record", "Playback"})  [unwired: 1 in]
        n291 = global write "WPI_DashboardLogging Global.vi" "Logging Filename"(path "") -> ()
        n292 = global write "WPI_DashboardLogging Global.vi" "Recording"(w477) -> ()
        n293 = case shown="\"Playback\"" w477 {
          tunnel: w476 -> [_ w479 w488]
          tunnel: [_ _ w487] -> w473
          tunnel: [_ _ w486] -> _
          tunnel: w471 -> [_ _ w484]
          tunnel: cluster{i32, i32} {-250, 170} -> [_ _ w483]
          tunnel: [_ _ T23 {"Image Size"=TRUE, "Image Type"=TRUE, "Pixel Value"=TRUE, "ROI Information"=TRUE, "Zoom Factor"=FALSE} ("Image Information Shown:All Elements")] -> w469
          tunnel: [_ _ TRUE ("Zoom Factor")] -> w468
          tunnel: w467 -> [_ _ w480]
          frame Default {
          }
          frame "Stop", "Record" {
            # "Place Window too"
            n294 = invoke class="VI" method="FP.Close"(reference=w479) -> (reference out=w478:refnum<vi>)  [unwired: 2 in, 2 out]
            n295 = invoke class="VI" method="Abort VI"(reference=w478) -> ()  [unwired: 2 in, 3 out]
          }
          frame "Playback" {
            n296 = call "Open Playback Panel.vi"("Offset"=w483, "DB VI Ref"=w484, "Playback in"=w488) -> ("Playback out"=w485:refnum<vi>)  [unwired: 8 in]
            n297 = register-events(w485, w480) -> (reference out=w487:refnum<event-registration>, error out=w486:errorcluster)  [unwired: 2 in]
          }
        }
        n298 = property on="Camera Image" class="ImageControl"("Image Information Shown"=w469, "Image Information Visible"=w468) -> ()  [unwired: 2 in, 2 out]
        n299 = call <vilib>:"WPI_DashboardNT Log FieldName Cache.vi"("Operation"=enum16{"Lookup/Add", "Index", "Clear"}."Clear") -> ()  [unwired: 8 in, 3 out]
      }
      event Panel Close {
        w490 = enum32{"Stop", "Record", "Playback"}."Stop" ("Rec Mode")
        # "Playback window has been closed, abort"
        n300 = event-data() -> ()  [unwired: 1 in, 4 out]
        n301 = local write "Rec Mode"(w490) -> ()
        n302 = global write "WPI_DashboardLogging Global.vi" "Recording"(w490) -> ()
      }
      event Panel Close {
        # "Abort playback window and ourself"
        n303 = event-data() -> ()  [unwired: 1 in, 4 out]
        n304 = invoke class="VI" method="FP.Close"(reference=w496) -> (reference out=w495:refnum<vi>)  [unwired: 2 in, 2 out]
        n305 = invoke class="VI" method="Abort VI"(reference=w495) -> (error out=w494:errorcluster)  [unwired: 2 in, 2 out]
        n306 = invoke class="VI" method="Abort VI"(error in=w494) -> ()  [unwired: 2 in, 3 out]
      }
      event User Event {
        n307 = event-data() -> ("IDs"=w504:cluster{"RPC field ID":u16, "Unique ID":u16}, "String"=w503:string)  [unwired: 1 in]
        n308 = Bundle("IDs"=w504, "String"=w503) -> (w502:T9)  [unwired: 1 in]
        n309 = call <vilib>:"Retrieve RPC Response.vi"("RPC Response"=w502) -> ("Output"=w499:string[][])  [unwired: 10 in]
        n310 = Build Array (concatenate)(w497, w499) -> (w498:string[][])
        n311 = local write "Command Params"(w498) -> ()
        n312 = local write "Cmd Status"("" ("Cmd Status")) -> ()
      }
      event "Vision": Value Change {
        # "Enable/Disable Compression slider.\nHW USB is hard-coded into the camera"
        n313 = event-data() -> ("NewVal"=w511:u16)  [unwired: 1 in]
        n314 = Equal?(x=w511, y=u32 2 ("milliseconds to wait")) -> (x = y?=w509:bool)
        n315 = Select(t=T24."Disabled and Grayed Out" ("Disabled"), s=w509, f=T24."Enabled" ("Disabled")) -> (s? t:f=w506:T24)
        n316 = property on="Compression" class="Slide (strict)"("DisabledEnum"=w506) -> ()  [unwired: 2 in, 2 out]
      }
      event "Tree": Double Click {
        n317 = event-data() -> ("PlatMods"=w516:T27, "Tag"=w515:string)  [unwired: 1 in]
        n318 = Unbundle(w516) -> ("Shift"=w514:bool)  [unwired: 4 out]
        n319 = Not(x=w514) -> (.not. x?=w513:bool)
        n320 = call <vilib>:"NT Update Persistence.vi"("Persistence"=w513, "Name"=w515) -> ()  [unwired: 9 in, 1 out]
      }
    }
  }
  n321 = while {
    tunnel: w47 -> [w520]
    i -> [w523]
    stop <- FALSE stop-if-true
    n322 = Wait (ms)(milliseconds to wait=u32 100) -> ()  [unwired: 1 out]
    n323 = case shown="\"Playback\"" "Rec Mode" {
      tunnel: w523 -> [_ _ w538]
      tunnel: [u32 2829099 ("Base Color") u32 11141120 ("Target Color") w527] -> w519
      frame "Stop", Default {
        # "Reset the color, extra updates don't cost much"
      }
      frame "Record" {
      }
      frame "Playback" {
        # "Playback"
        n324 = Quotient & Remainder(x=w538, y=u32 50 ("milliseconds to wait")) -> (x-y*floor(x/y)=w534:u32)  [unwired: 1 out]
        n325 = Divide(x=w534, y=u32 50 ("milliseconds to wait")) -> (x/y=w531:dbl)
        n326 = Multiply(x=6.283185307179586, y=w531) -> (x*y=w536:dbl)
        n327 = Sine(x=w536) -> (sin(x)=w535:dbl)
        n328 = Absolute Value(x=w535) -> (abs(x)=w528:dbl)
        n329 = call "Interpolate RGB Color.vi"("Proportion"=w528, "Target Color"=u32 30976, "Base Color"=u32 2829099) -> ("Result Color"=w527:u32)  [unwired: 8 in]
      }
    }
    n330 = property class="Pane"(reference=w520, "PaneColor"=w519) -> ()  [unwired: 1 in, 2 out]
  }
  n331 = local write "Dashboard Tab"(T1."Drive" ("Dashboard Tab")) -> ()
  n332 = property on="On/Off" class="Bool (strict)"("Visible"=w15) -> ()  [unwired: 2 in, 2 out]
  n333 = property on="Motor" class="Clust (strict)"("Visible"=w15) -> ()  [unwired: 2 in, 2 out]
  n334 = property on="Progress" class="Clust (strict)"("Visible"=w15) -> ()  [unwired: 2 in, 2 out]
  n335 = property on="Test Ring" class="Ring (strict)"("Visible"=w15) -> ()  [unwired: 2 in, 2 out]
  n336 = property on="Rev/Fwd" class="Clust (strict)"("Visible"=w15) -> ()  [unwired: 2 in, 2 out]
  n337 = property on="Camera Settings" class="Clust (strict)"("Visible"=w15) -> ()  [unwired: 2 in, 2 out]
  n338 = while {
    tunnel: u16 1741 ("timeout ms (25000)") -> [w540]
    stop <- FALSE stop-if-true
    n339 = TCP Create Listener(10:w540) -> (0:w539:errorcluster, 3:w541:refnum<k5>)  [unwired: 4 in, 1 out]
    n340 = case shown="No Error" w539 {
      selector: w539 -> [w543 _]
      tunnel: w541 -> [w544 _]
      frame No Error {
        n341 = while {
          tunnel: w544 -> [w547]
          tunnel: w543 -> [w546]
          stop <- FALSE stop-if-true
          n342 = TCP Wait On Listener(8:w546, 11:w547) -> (0:w548:errorcluster, 4:w549:refnum<k5>)  [unwired: 2 in, 3 out]
          n343 = local write "TCP"(w549) -> ()
          n344 = case shown="No Error" w548 {
            frame No Error {
            }
            frame Error {
              n345 = Wait (ms)(milliseconds to wait=u32 1000) -> ()  [unwired: 1 out]
            }
          }
        }
      }
      frame Error {
        n346 = Wait (ms)(milliseconds to wait=u32 1000) -> ()  [unwired: 1 out]
      }
    }
  }
  n347 = local write "DB Camera Config"(w15) -> ()
  n348 = local write "Command Params"(string[][] [] ("Command Params")) -> ()
  n349 = global write "WPI_DashboardLogging Global.vi" "Recording"(w41) -> ()
  n350 = local write "Command Selection"(u16 0 ("milliseconds to wait")) -> ()
  n351 = local write "Rec Mode"(w41) -> ()
